vi "create_task.vi"(8 "error in":errorcluster, 10 "NP":tag="PXI1Slot4_2" caption="Nome da placa", 11 "ClusterIn":T1={"Simulation?"=FALSE, "ChanConfigs"=[], "Essay Config"={"HoleDiam"=1.4, "MeanLineDiam"=5.0, "IncF"=0.2, "ElastMod"=207.0, "PoissonMod"=0.3, "RosType"=enum."Tipo A", "Método de análise"=enum."Simplificado 2008", "Pfinal"=0.3, "AStop"=TRUE}, "Directory"=path "", "EssayName"="", "RawFile"=refnum, "InfoFile"=refnum, "DataFile"=refnum, "task"="", "qRecord"=refnum, "qProcess"=refnum} {"ChanConfigs"."GF" min=0.1 max=10.0; "ChanConfigs"."Canal" min=1 max=8}) -> (0 "error out":errorcluster, 3 "Cluster":T1={"Simulation?"=FALSE, "ChanConfigs"=[], "Essay Config"={"HoleDiam"=1.4, "MeanLineDiam"=5.0, "IncF"=0.2, "ElastMod"=207.0, "PoissonMod"=0.3, "RosType"=enum."Tipo A", "Método de análise"=enum."Simplificado 2008", "Pfinal"=0.3, "AStop"=TRUE}, "Directory"=path "", "EssayName"="", "RawFile"=refnum, "InfoFile"=refnum, "DataFile"=refnum, "task"="", "qRecord"=refnum, "qProcess"=refnum} {"ChanConfigs"."GF" min=0.1 max=10.0; "ChanConfigs"."Canal" min=1 max=8})   [LabVIEW 2016]
uses:
  MainFGV/cluster_main_FGV.ctl
  Channel_config.ctl
  essay_config.ctl
  <vilib>/DAQmx/create/channels.llb/DAQmx Create Channel (AI-Strain-Strain Gage).vi
  <vilib>/DAQmx/calibration/calibrationInfo.llb/DAQmx Perform Shunt Calibration Ex (Strain).vi
  <vilib>/DAQmx/configure/timing.llb/DAQmx Timing (Sample Clock).vi
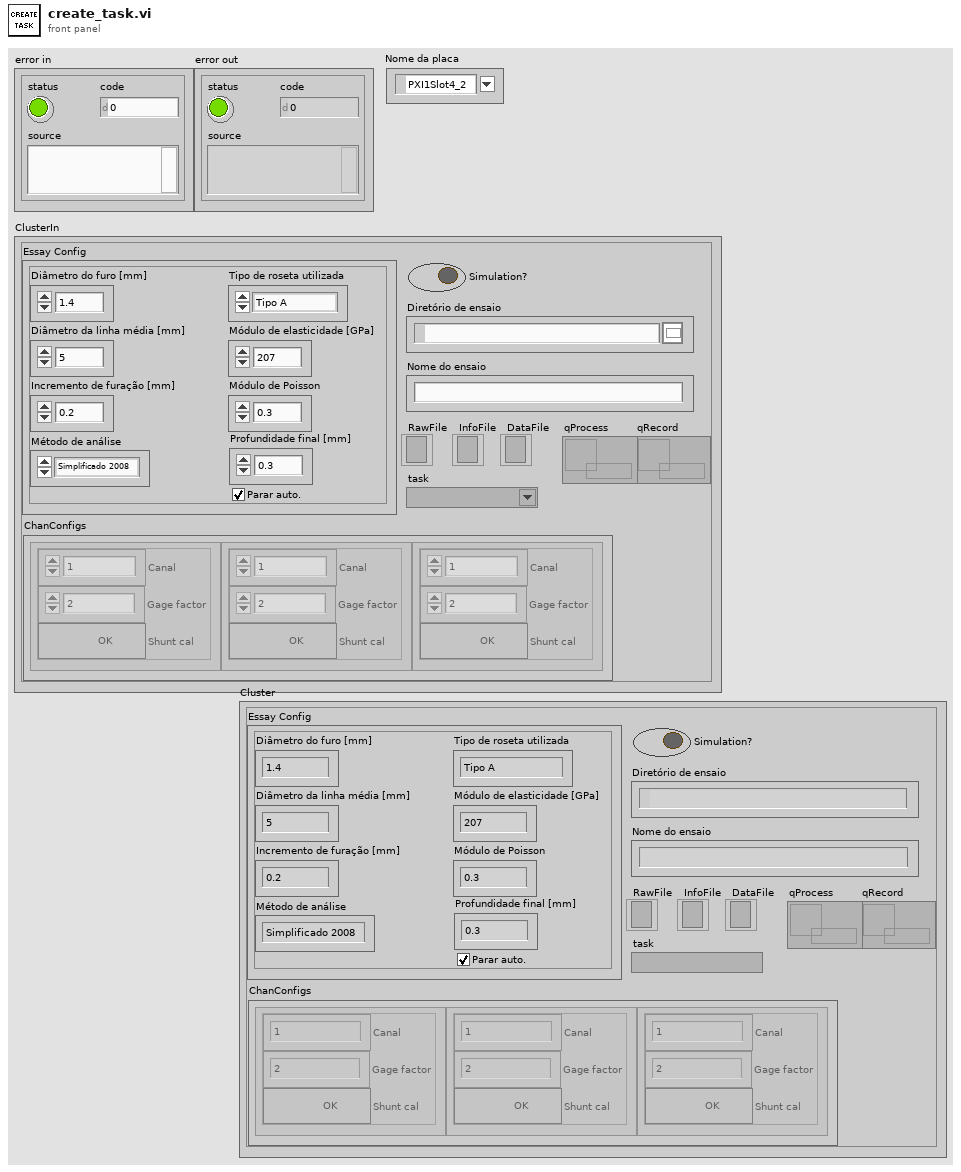
[diagram p1: front panel]
types:
  T1 = typedef "cluster_main_FGV.ctl" = cluster{"Simulation?":bool, "ChanConfigs":T2[], "Essay Config":T3, "Directory":path, "EssayName":string, "RawFile":refnum<file>, "InfoFile":refnum<file>, "DataFile":refnum<file>, "task":refnum<k21>, "qRecord":refnum<queue>, "qProcess":refnum<queue>}
  T2 = typedef "Channel_config.ctl" = cluster{"Canal":i32, "GF":dbl, "SC":bool}
  T3 = typedef "essay_config.ctl" = cluster{"HoleDiam":dbl, "MeanLineDiam":dbl, "IncF":dbl, "ElastMod":dbl, "PoissonMod":dbl, "RosType":enum16{"Tipo A", "Tipo B", "Tipo C"}, "Método de análise":enum16{"Não uniforme 2013", "Simplificado 2013", "Simplificado 2008"}, "Pfinal":dbl, "AStop":bool}
  T4 = cluster{"gage factor":dbl, "nominal gage resistance":dbl, "poisson ratio":dbl}
  T5 = cluster{"strain configuration":i32, "lead wire resistance":dbl, "initial bridge voltage":dbl, "voltage excitation source":i32, "voltage excitation value":dbl}
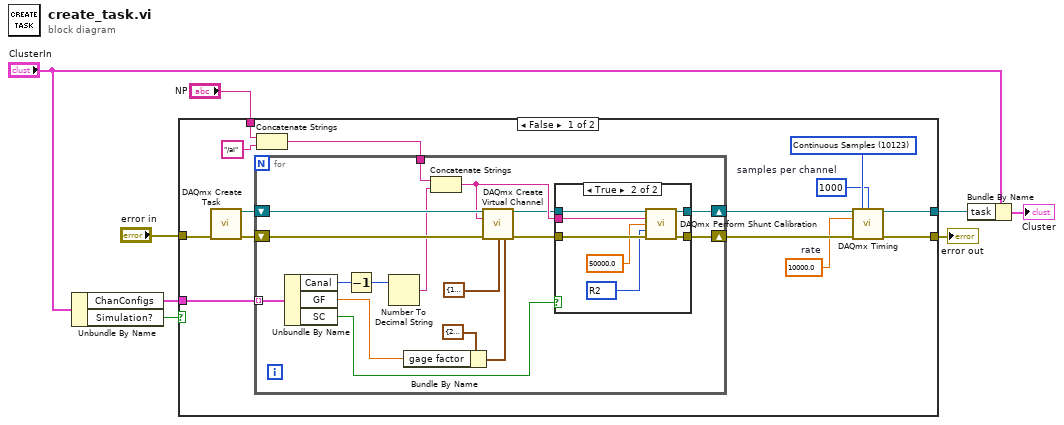
[diagram p0: block diagram]
diagram:
  n1 = Unbundle By Name("ClusterIn") -> ("ChanConfigs"=w5:T2[], "Simulation?"=w4:bool)
  n2 = case shown="False" w4 {
    tunnel: w5 -> [w15 _]
    tunnel: [w14 w49] -> w6
    tunnel: [w13 _] -> w2
    tunnel: "NP" -> [w12 _]
    tunnel: "error in" -> [w9 w49]
    frame False {
      w10 = 1000  # samples per channel
      w11 = 10000.0  # rate
      w16 = 10123 items=["Finite Samples"=10178, "Continuous Samples"=10123, "Hardware Timed Single Point"=12522] ("sample mode")
      n3 = call <vilib>:"DAQmx Create Task.vi"("error in"=w9) -> ("task out"=w22:refnum<k21>, "error out"=w21:errorcluster)  [unwired: 13 in]
      n4 = Concatenate Strings(w12, "/ai" ("string")) -> (w19:string)
      n5 = for {
        tunnel: w15 -> [w34] mode=indexing
        shift-right: [w37] -> w17
        shift-left: w21 -> [w39]
        tunnel: w19 -> [w36]
        shift-right: [w35] -> w18
        shift-left: w22 -> [w38]
        n6 = Unbundle By Name(w34) -> ("Canal"=w25:i32, "GF"=w31:dbl, "SC"=w29:bool)
        n7 = Decrement(x=w25) -> (x-1=w24:i32)
        n8 = Number To Decimal String(number=w24) -> (decimal integer string=w23:string)  [unwired: 1 in]
        n9 = Bundle By Name(cluster=T4 {"gage factor"=2.0, "nominal gage resistance"=120.0, "poisson ratio"=0.3} ("strain gage information"), "gage factor"=w31) -> (w32:T4)
        n10 = Concatenate Strings(w36, w23) -> (w30:string)
        n11 = call-poly <vilib>:"DAQmx Create Virtual Channel.vi"("task in"=w38, "physical channels"=w30, "error in"=w39, "bridge information"=T5 {"strain configuration"=10271, "lead wire resistance"=0.0, "initial bridge voltage"=0.0, "voltage excitation source"=10200, "voltage excitation value"=2.0}, "strain gage information"=w32) -> ("task out"=w26:refnum<k21>, "error out"=w27:errorcluster)  [unwired: 9 in]
        n12 = case shown="True" w29 {
          tunnel: w26 -> [w41 w48]
          tunnel: [w41 w47] -> w35
          tunnel: w27 -> [w40 w46]
          tunnel: [w40 w45] -> w37
          tunnel: w30 -> [_ w44]
          frame False {
          }
          frame True {
            w43 = 12466 items=["R1"=12465, "R2"=12466, "R3"=12467, "R4"=14813] ("shunt element location")
            n13 = call-poly <vilib>:"DAQmx Perform Shunt Calibration.vi"("task/channels in"=w48, "channels"=w44, "shunt resistance"=50000.0, "shunt element location"=w43, "error in"=w46) -> ("task out"=w47:refnum<k21>, "error out"=w45:errorcluster)  [unwired: 9 in]
          }
        }
      }
      n14 = call-poly <vilib>:"DAQmx Timing.vi"("task/channels in"=w18, "sample mode"=w16, "samples per channel"=w10, "rate"=w11, "error in"=w17) -> ("task out"=w13:refnum<k21>, "error out"=w14:errorcluster)  [unwired: 9 in]
    }
    frame True {
    }
  }
  "error out" <- w6
  n15 = Bundle By Name(cluster="ClusterIn", "task"=w2) -> (→"Cluster":T1)
